vi "start.vi"(8 "error in (no error)":errorcluster, 11 "ExperimentControllerDL090130Interval in":refnum<class "ExperimentControllerDL090130Interval.lvclass">) -> (0 "error out":errorcluster, 3 "ExperimentControllerDL090130Interval out":refnum<class "ExperimentControllerDL090130Interval.lvclass">)   [LabVIEW 2010, in "ExperimentControllerDL090130Interval.lvclass"]
uses:
  ExperimentControllerDL090130Interval.lvclass
  schedule_entry_cluster.ctl
  internal_trigger_enum.ctl
  ExperimentControllerDL090130Interval.lvclass/ExperimentControllerDL090130Interval.ctl
  common/classes/ErrorController/ErrorController/class_data.vi
  common/classes/ErrorController/ErrorController/ErrorController.lvclass
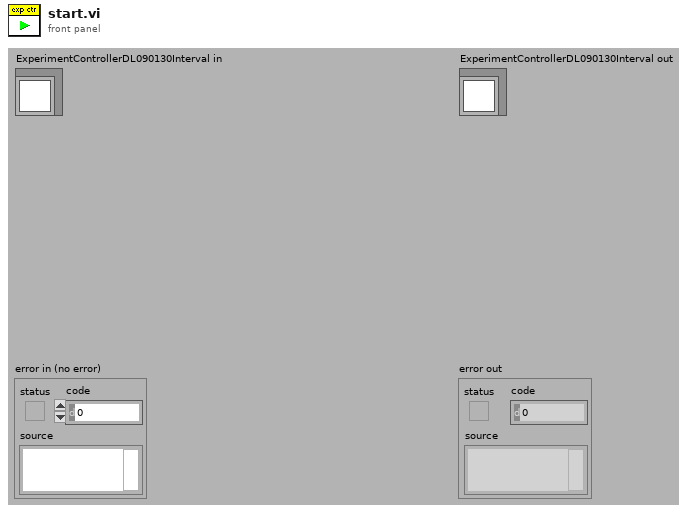
[diagram p1: front panel]
types:
  T1 = typedef "ExperimentControllerDL090130Interval.lvclass/schedule_entry_cluster.ctl" = cluster{"time":timestamp, "trigger":T2}
  T2 = typedef "ExperimentControllerDL090130Interval.lvclass/internal_trigger_enum.ctl" = enum16{"NULL", "initialise", "terminate", "start", "stop", "proceed", "prepare", "start sweep"}
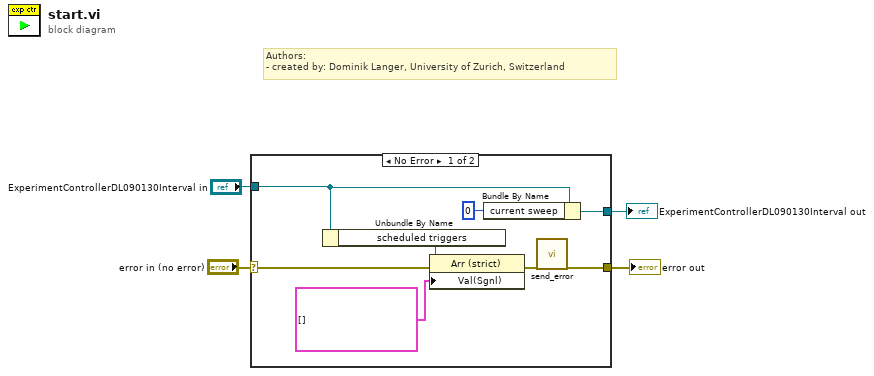
[diagram p0: block diagram]
diagram:
  # "Authors: \n- created by: Dominik Langer, University of Zurich, Switzerland"
  n1 = case shown="No Error" "error in (no error)" {
    selector: "error in (no error)" -> [w10 w14]
    tunnel: [w5 w14] -> w4
    tunnel: [w12 w13] -> w3
    tunnel: "ExperimentControllerDL090130Interval in" -> [w8 w13]
    frame No Error {
      n2 = Unbundle By Name(w8) -> ("scheduled triggers"=w11:refnum<vi>)
      n3 = property class="Arr (strict)"(reference=w11, error in=w10, "Val(Sgnl)"=T1[] [] ("Value (Signaling)")) -> (error out=w6:errorcluster)  [unwired: 1 out]
      n4 = Bundle By Name(cluster=w8, "current sweep"=0) -> (w12:refnum<class "ExperimentControllerDL090130Interval.lvclass">)
      n5 = call "send_error.vi"("error in (no error)"=w6) -> ("error out"=w5:errorcluster)  [unwired: 10 in]
    }
    frame Error {
    }
  }
  "error out" <- w4
  "ExperimentControllerDL090130Interval out" <- w3
